vi "Check Status No Objects - Fluke Multimeter.vi"(8 "error in (no error)":errorcluster, 10 "VISA Resource Name":refnum<visa-resource-name>="GPIB0::2::INSTR", 11 "input cluster":T1) -> (0 "error out":errorcluster, 1 "Status":string, 2 "Ready?":bool, 3 "output cluster":T1)   [LabVIEW 2012]
doc: "(Dynamic) Check if the instrument is powered on and update its member data with the instrument's current status. Optionally return a text status message."
uses:
  Fluke 8840/Fluke 8840.lvlib
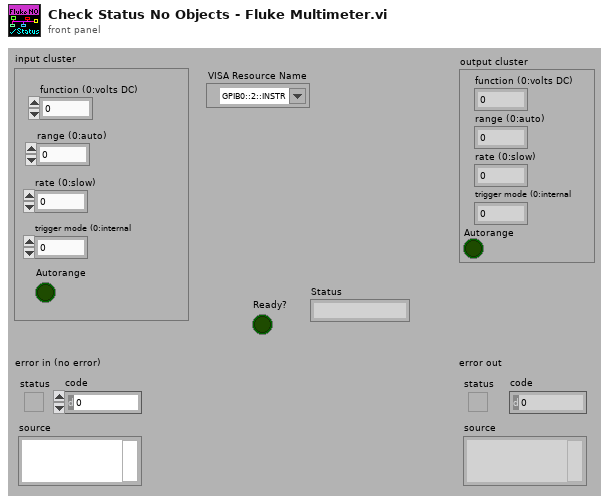
[diagram p1: front panel]
types:
  T1 = cluster{"function (0:volts DC)":i16, "range (0:auto)":i16, "rate (0:slow)":i16, "trigger mode (0:internal":i16, "Autorange":bool}
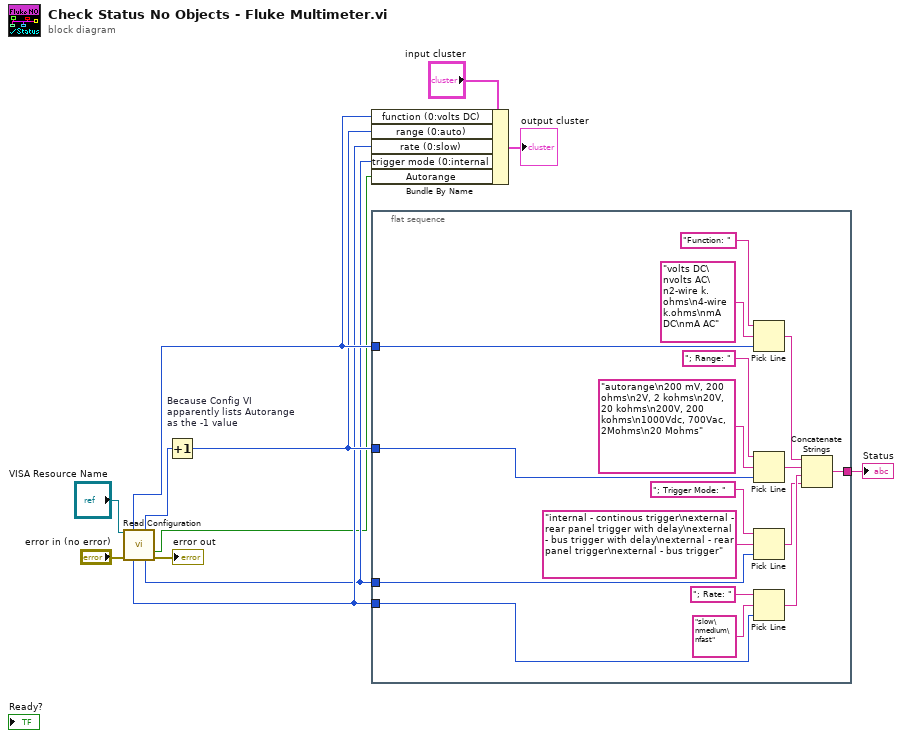
[diagram p0: block diagram]
diagram:
  n1 = call "Read Configuration.vi"("VISA resource name"="VISA Resource Name", "error in (no error)"="error in (no error)") -> ("function"=w10:i32, "range"=w11:i32, "autorange"=w6:bool, "rate"=w8:i32, "trigger mode"=w7:i32, "error out"=→"error out":errorcluster)  [unwired: 8 out]
  n2 = Increment "Because Config VI\napparently lists Autorange\nas the -1 value"(x=w11) -> (x+1=w9:i32)
  n3 = Bundle By Name(cluster="input cluster", "function (0:volts DC)"=w10, "range (0:auto)"=w9, "rate (0:slow)"=w8, "trigger mode (0:internal"=w7, "Autorange"=w6) -> (→"output cluster":T1)
  n4 = flat-sequence {
    tunnel: [w27] -> w12
    tunnel: w10 -> [w25]
    tunnel: w9 -> [w22]
    tunnel: w8 -> [w17]
    tunnel: w7 -> [w16]
    frame #0 {
      n5 = Pick Line(string ("")="Function: ", multi-line string="volts DC\nvolts AC\n2-wire k.ohms\n4-wire k.ohms\nmA DC\nmA AC", line index=w25) -> (output string=w28:string)
      n6 = Pick Line(string ("")="; Range: ", multi-line string="autorange\n200 mV, 200 ohms\n2V, 2 kohms\n20V, 20 kohms\n200V, 200 kohms\n1000Vdc, 700Vac, 2Mohms\n20 Mohms", line index=w22) -> (output string=w21:string)
      n7 = Pick Line(string ("")="; Trigger Mode: ", multi-line string="internal - continous trigger\nexternal - rear panel trigger with delay\nexternal - bus trigger with delay\nexternal - rear panel trigger\nexternal - bus trigger", line index=w16) -> (output string=w13:string)
      n8 = Pick Line(string ("")="; Rate: ", multi-line string="slow\nmedium\nfast", line index=w17) -> (output string=w14:string)
      n9 = Concatenate Strings(w28, w21, w14, w13) -> (w27:string)
    }
  }
  "Status" <- w12
